vi "set_vacuum.vi"(0 "Remote":bool, 1 "Atm":bool, 2 "Vac Exhaust":bool) -> ()   [LabVIEW 2011]
uses:
  low_level_proc/globals.vi
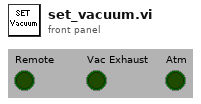
[diagram p1: front panel]
types:
  T1 = typedef "relaySpec.ctl" = cluster{"Card Index":u16, "Relay Index":u16}
  T2 = cluster{"Relay Functions":cluster{"Remote":T1, "Atm":T1, "Exhaust":T1}}
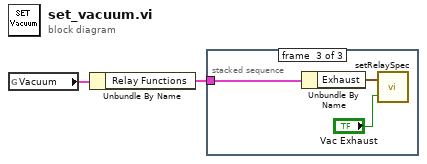
[diagram p0: block diagram]
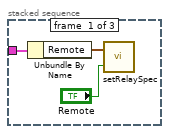
[diagram p2: hidden frame]
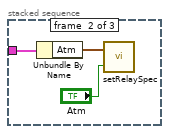
[diagram p3: hidden frame]
diagram:
  n1 = global read "globals.vi" "Vacuum"() -> (w2:T2)
  n2 = Unbundle By Name(w2) -> ("Relay Functions"=w1:cluster{"Remote":T1, "Atm":T1, "Exhaust":T1})
  n3 = stacked-sequence {
    tunnel: w1 -> [w5 w7 w10]
    frame #0 {
      n4 = Unbundle By Name(w5) -> ("Remote"=w3:T1)
      n5 = call "setRelaySpec.vi"("Relay Status"="Remote", "RelaySpec"=w3) -> ()  [unwired: 1 in]
    }
    frame #1 {
      n6 = Unbundle By Name(w7) -> ("Atm"=w6:T1)
      n7 = call "setRelaySpec.vi"("Relay Status"="Atm", "RelaySpec"=w6) -> ()  [unwired: 1 in]
    }
    frame #2 {
      n8 = Unbundle By Name(w10) -> ("Exhaust"=w9:T1)
      n9 = call "setRelaySpec.vi"("Relay Status"="Vac Exhaust", "RelaySpec"=w9) -> ()  [unwired: 1 in]
    }
  }
